vi "To Pythonic - Boolean.vi"(4 "Boolean":bool) -> (1 "Pythonic Value":string)   [LabVIEW 2012, in "OPI.lvclass"]
doc: "Convert LabVIEW data into valid pythonic representation."
uses:
  OPI.lvclass
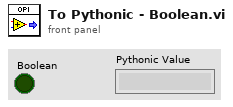
[diagram p1: front panel]
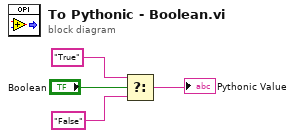
[diagram p0: block diagram]
diagram:
  n1 = Select(t="True", s="Boolean", f="False") -> (s? t:f=→"Pythonic Value":string)
